vi "Status_Log.vi"(8 "error in (no error)":errorcluster, 10 "String":string, 11 "Status Queue":refnum<queue>) -> (0 "error out":errorcluster)   [LabVIEW 2015]
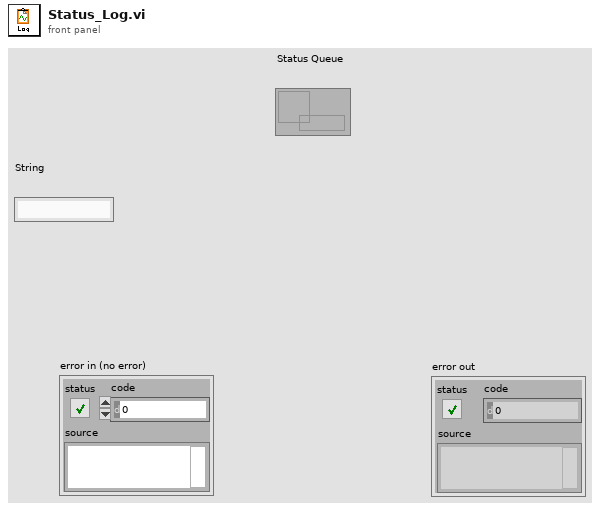
[diagram p1: front panel]
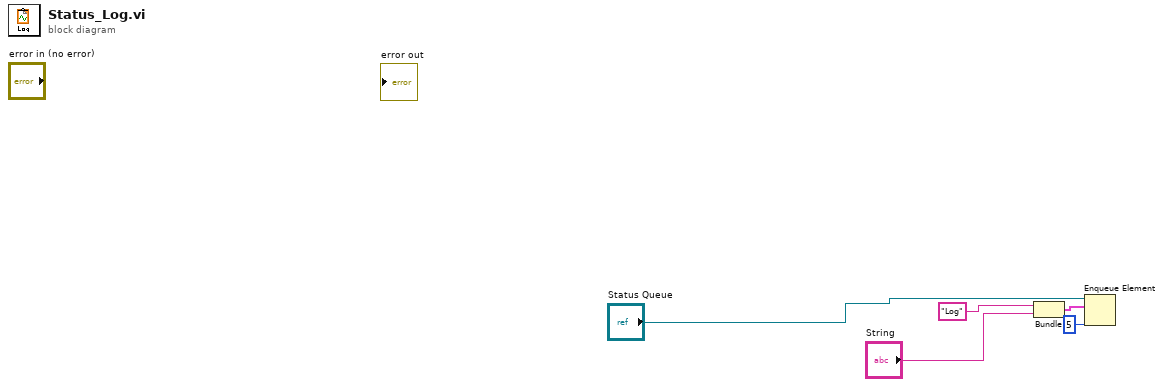
[diagram p0: block diagram]
diagram:
  n1 = Bundle("Log", "String"="String") -> (w5:cluster{string, "String":string})  [unwired: 1 in]
  n2 = Enqueue Element(queue="Status Queue", element=w5, timeout in ms (-1)=5) -> ()  [unwired: 1 in, 3 out]
